vi "Read Name for CMenu.vi"(8 "error in (no error)":errorcluster, 11 "Analyze BaseClass in":refnum<class "Analyze BaseClass.lvclass">) -> (0 "error out":errorcluster, 2 "Name for Context menu":string, 3 "Analyze BaseClass out":refnum<class "Analyze BaseClass.lvclass">)   [LabVIEW 2020, in "Analyze.lvlib" / "Analyze BaseClass.lvclass"]
uses:
  Analyze BaseClass.lvclass
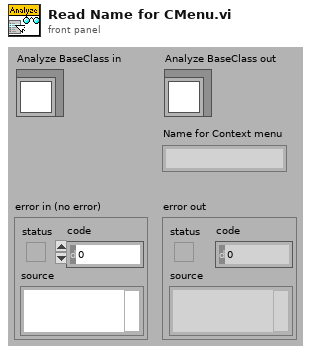
[diagram p1: front panel]
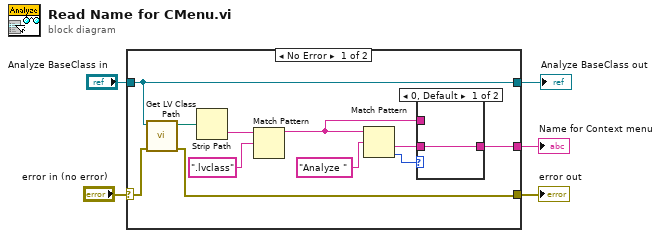
[diagram p0: block diagram]
diagram:
  n1 = case shown="No Error" "error in (no error)" {
    selector: "error in (no error)" -> [w15 w20]
    tunnel: [w14 w20] -> w4
    tunnel: [w16 w19] -> w2
    tunnel: "Analyze BaseClass in" -> [w16 w19]
    tunnel: [w8 _] -> w1
    frame No Error {
      n2 = call <vilib>:"Get LV Class Path.vi"("error in (no error)"=w15, "object"=w16) -> ("error out"=w14:errorcluster, "class path"=w13:path)  [unwired: 8 in]
      n3 = Strip Path(path=w13) -> (name=w11:string)  [unwired: 1 out]
      n4 = Match Pattern(string=w11, regular expression=".lvclass" ("search string/char (-)")) -> (before substring=w6:string)  [unwired: 1 in, 3 out]
      n5 = Match Pattern(string=w6, regular expression="Analyze ") -> (after substring=w7:string, offset past match=w9:i32)  [unwired: 1 in, 2 out]
      n6 = case shown="0, Default" w9 {
        tunnel: [w17 w18] -> w8
        tunnel: w7 -> [w17 _]
        tunnel: w6 -> [_ w18]
        frame 0, Default {
        }
        frame -1 {
        }
      }
    }
    frame Error {
    }
  }
  "error out" <- w4
  "Analyze BaseClass out" <- w2
  "Name for Context menu" <- w1
